vi "ADS5463模块换算.vi"(1 "ADC最小电压":dbl, 2 "ADC最大电压":dbl, 3 "ADC精度":u16, 4 "16进制返回值":u16) -> (0 "实际电压":dbl)   [LabVIEW 2017]
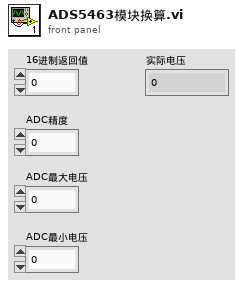
[diagram p1: front panel]
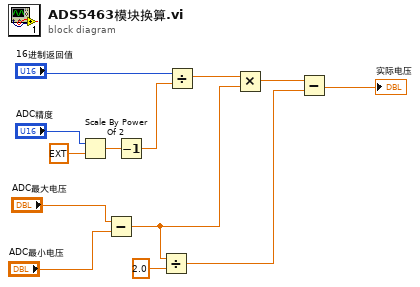
[diagram p0: block diagram]
diagram:
  n1 = Scale By Power Of 2(n="ADC精度", x=ext 1.0) -> (x*2^n=w11:ext)
  n2 = Subtract(x="ADC最大电压", y="ADC最小电压") -> (x-y=w5:dbl)
  n3 = Decrement(x=w11) -> (x-1=w9:ext)
  n4 = Divide(x=w5, y=2.0) -> (x/y=w2:dbl)
  n5 = Divide(x="16进制返回值", y=w9) -> (x/y=w8:ext)
  n6 = Multiply(x=w8, y=w5) -> (x*y=w3:ext)
  n7 = Subtract(x=w3, y=w2) -> (x-y=→"实际电压":ext)
